vi "263-264-2.vi"() -> ()   [LabVIEW 2020]
uses:
  C:/Program Files (x86)/National Instruments/LabVIEW 2020/examples/Connectivity/Python/support/PythonVersionsEnum.ctl
panel:
  out "时间字符串 2":string
  out "时间字符串":string
  out "连接的字符串 2":string
  out "连接的字符串":string
  out "字符串":string
  out "error out 2":cluster{"状态":bool, "代码":i32, "源":string} caption="错误输出"
  out "非压缩地址 2":string
  out "压缩地址 2":string
  in  "error in (no error)":cluster{"状态":bool, "代码":i32, "源":string} caption="错误输入（无错误）"
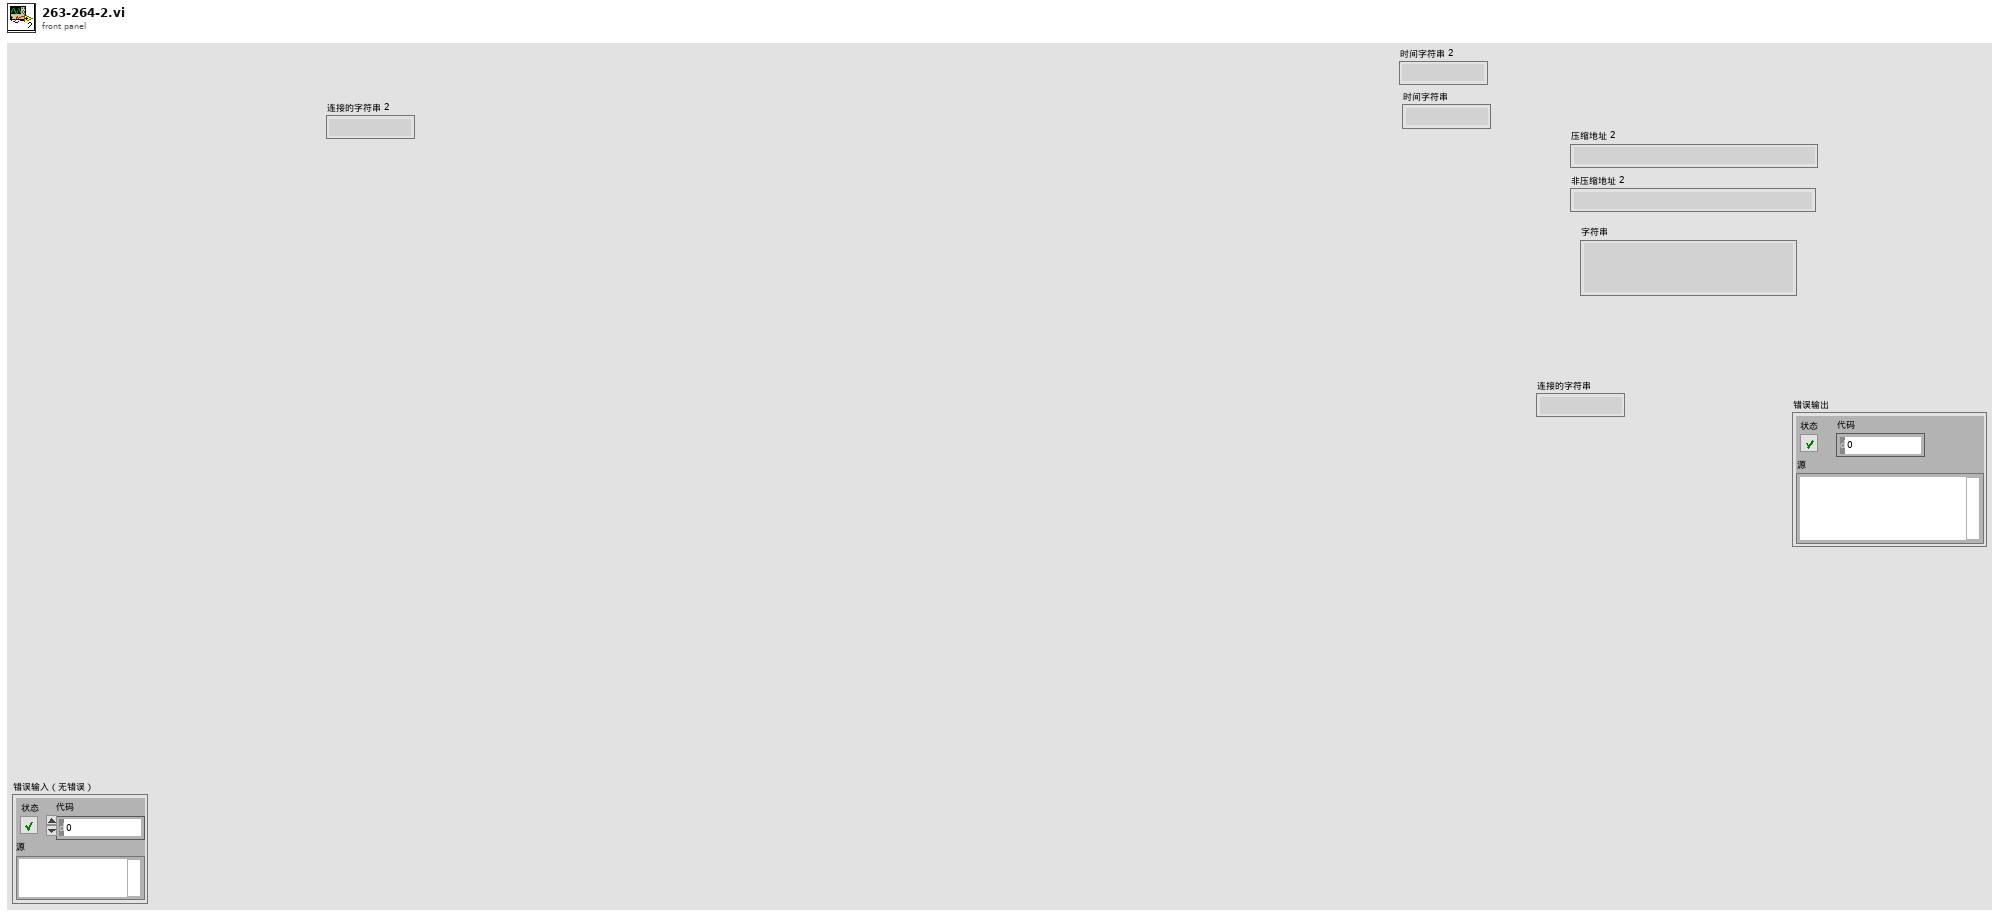
[diagram p1: front panel]
types:
  T1 = typedef "PythonVersionsEnum.ctl" = enum16{"2.7", "3.6"}
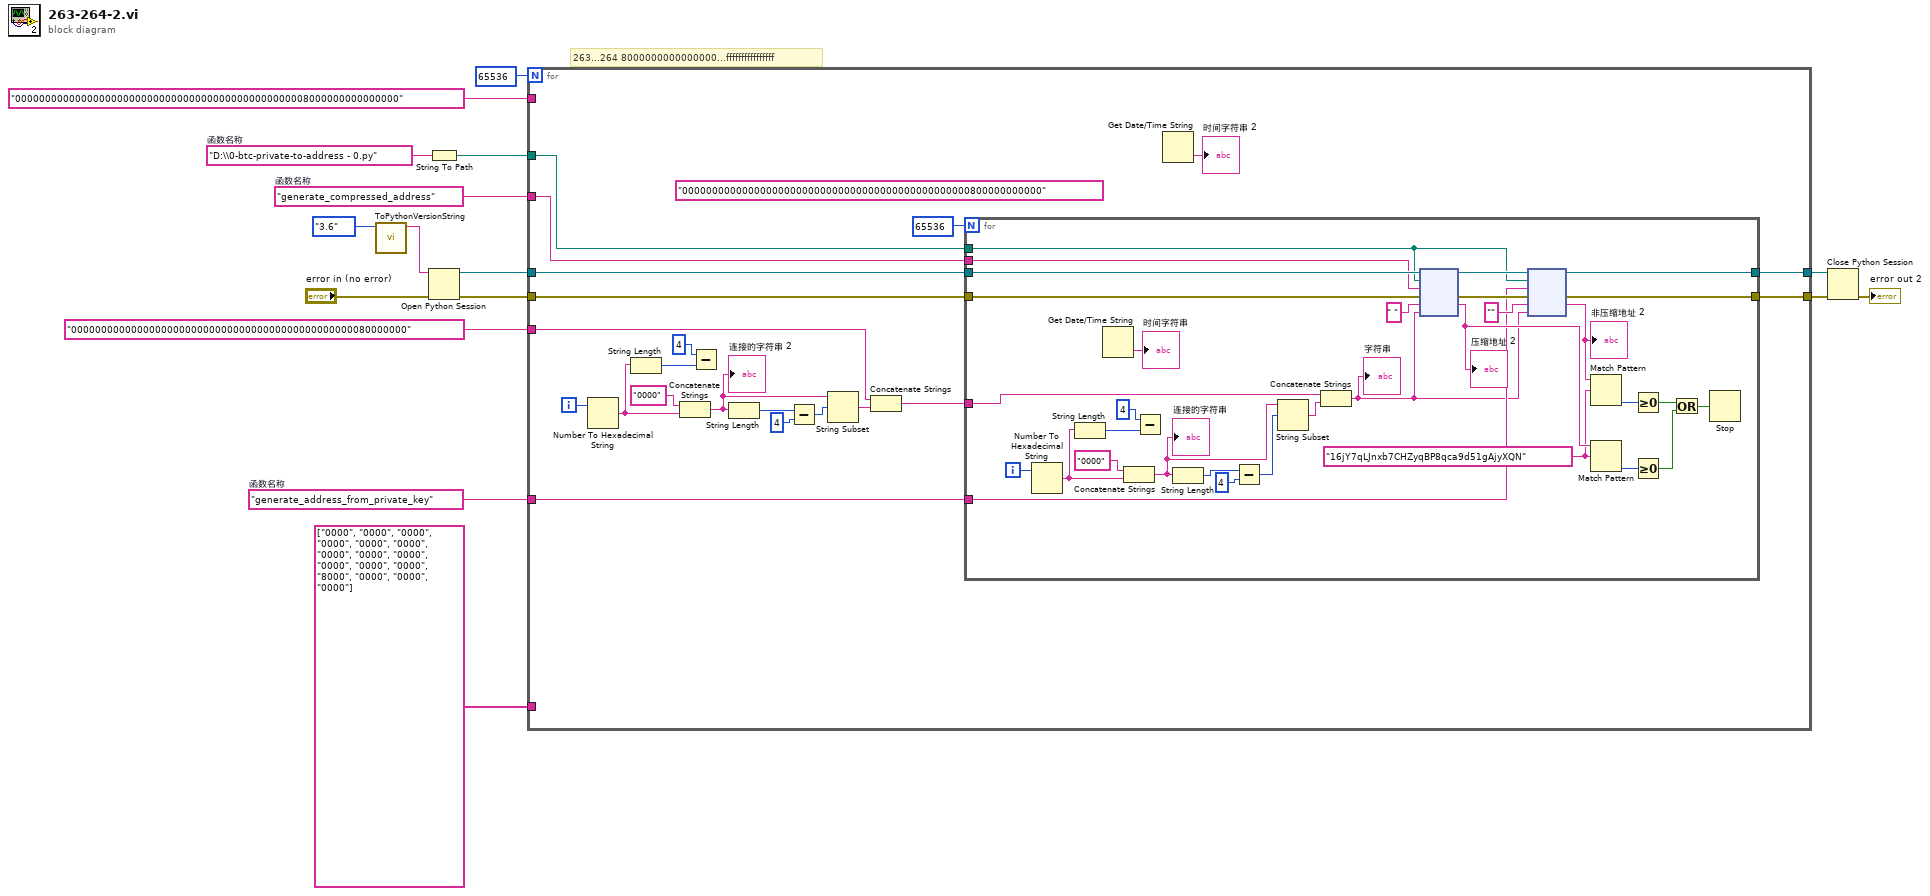
[diagram p0: block diagram]
diagram:
  w4 = "generate_compressed_address"  # 函数名称
  w6 = "D:\\0-btc-private-to-address - 0.py"  # 函数名称
  w7 = "generate_address_from_private_key"  # 函数名称
  # "263...264\t8000000000000000...ffffffffffffffff"
  n1 = call "ToPythonVersionString.vi"("Python版本"=PythonVersionsEnum."3.6") -> ("python版本字符串"=w15:string)  [unwired: 10 in]
  n2 = String To Path(string=w6) -> (path=w5:path)
  n3 = Open Python Session(python version=w15, 3:"error in (no error)") -> (session out=w12:refnum<k35>, error out=w11:errorcluster)  [unwired: 1 in]
  n4 = for {
    N: 65536 -> [_]
    tunnel: string[] ["0000", "0000", "0000", "0000", "0000", "0000", "0000", "0000", "0000", "0000", "0000", "0000", "8000", "0000", "0000", "0000"] ("数组") -> [_]
    tunnel: w12 -> [w36]
    tunnel: w11 -> [w35]
    tunnel: [w34] -> w9
    tunnel: [w33] -> w8
    tunnel: w7 -> [w32]
    tunnel: w5 -> [w31]
    tunnel: w4 -> [w30]
    tunnel: "0000000000000000000000000000000000000000000000008000000000000000" ("字符串 3") -> [_]
    tunnel: "00000000000000000000000000000000000000000000000080000000" ("字符串 3") -> [w19]
    i -> [w20]
    (unwired) "000000000000000000000000000000000000000000000000800000000000" ("字符串 3")
    n5 = Number To Hexadecimal String(2:w20) -> (0:w26:string)  [unwired: 1 in]
    n6 = String Length(string=w26) -> (length=w29:i32)
    n7 = Concatenate Strings("0000", w26) -> (w25:string)
    "连接的字符串 2" <- w25
    n8 = Subtract(x=4 ("y"), y=w29) -> ()  [unwired: 1 out]
    n9 = String Length(string=w25) -> (length=w23:i32)
    n10 = Subtract(x=w23, y=4) -> (x-y=w24:i32)
    n11 = String Subset(string=w25, offset (0)=w24) -> (substring=w21:string)  [unwired: 1 in]
    n12 = Concatenate Strings(w19, w21) -> (w18:string)
    n13 = for {
      N: 65536 -> [_]
      tunnel: w36 -> [w62]
      tunnel: w35 -> [w61]
      tunnel: [w60] -> w34
      tunnel: [w59] -> w33
      tunnel: w32 -> [w51]
      tunnel: w31 -> [w50]
      tunnel: w30 -> [w49]
      tunnel: w18 -> [w40]
      i -> [w67]
      w48 = "16jY7qLJnxb7CHZyqBP8qca9d51gAjyXQN"
      n14 = Number To Hexadecimal String(2:w67) -> (0:w46:string)  [unwired: 1 in]
      n15 = String Length(string=w46) -> (length=w69:i32)
      n16 = Get Date/Time String() -> (time string=→"时间字符串":string)  [unwired: 3 in, 1 out]
      n17 = Concatenate Strings("0000", w46) -> (w45:string)
      "连接的字符串" <- w45
      n18 = Subtract(x=4 ("y"), y=w69) -> ()  [unwired: 1 out]
      n19 = String Length(string=w45) -> (length=w43:i32)
      n20 = Subtract(x=w43, y=4) -> (x-y=w44:i32)
      n21 = String Subset(string=w45, offset (0)=w44) -> (substring=w41:string)  [unwired: 1 in]
      n22 = Concatenate Strings(w40, w41) -> (w39:string)
      "字符串" <- w39
      n23 = node(w62, w50, w49, w61, " ", w39) -> (w66:refnum<k35>, w65:errorcluster, w58:string)  [unwired: 1 in, 2 out]
      "压缩地址 2" <- w58
      n24 = node(w66, w50, w51, w65, "", w39) -> (w60:refnum<k35>, w59:errorcluster, w57:string)  [unwired: 1 in, 2 out]
      "非压缩地址 2" <- w57
      n25 = Match Pattern(string=w57, regular expression=w48) -> (offset past match=w56:i32)  [unwired: 1 in, 3 out]
      n26 = Match Pattern(string=w58, regular expression=w48) -> (offset past match=w55:i32)  [unwired: 1 in, 3 out]
      n27 = Greater Or Equal To 0?(x=w56) -> (x >= 0?=w54:bool)
      n28 = Greater Or Equal To 0?(x=w55) -> (x >= 0?=w53:bool)
      n29 = Or(x=w54, y=w53) -> (x .or. y?=w52:bool)
      n30 = Stop(stop? (T)=w52) -> ()
    }
    n31 = Get Date/Time String() -> (time string=→"时间字符串 2":string)  [unwired: 3 in, 1 out]
  }
  n32 = Close Python Session(session in=w9, error in=w8) -> (11:→"error out 2":errorcluster)
